vi "Apply.vi"(8 "Error In":errorcluster, 11 "Acquire Continuous Waveform CFG":refnum<class "Continuous Waveform Acq CFG.lvclass">) -> (0 "Error Out":errorcluster, 3 "Acquire Continuous Waveform CFG out":refnum<class "Continuous Waveform Acq CFG.lvclass">)   [LabVIEW 2023, in "RIGOL DS1054.lvlib" / "Continuous Waveform Acq CFG.lvclass"]
uses:
  Continuous Waveform Acq CFG.lvclass
  Continuous Waveform Acq CFG.lvclass/Continuous Waveform Acq CFG.ctl
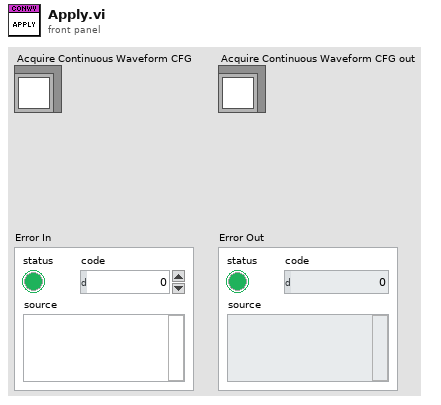
[diagram p1: front panel]
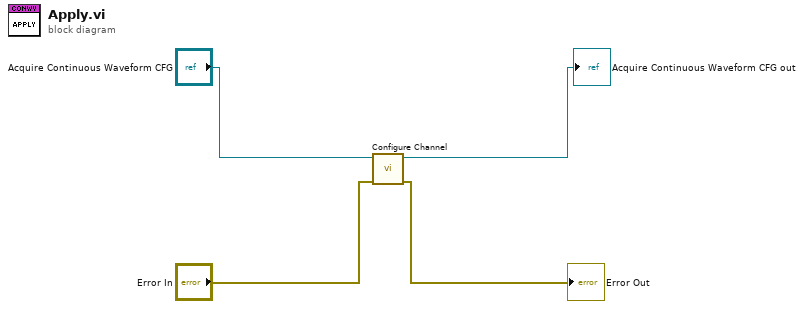
[diagram p0: block diagram]
diagram:
  n1 = call-dynamic "Configure Channel.vi"("error in"="Error In", "Continuous Waveforn Acq CFG in"="Acquire Continuous Waveform CFG") -> ("error out"=→"Error Out":errorcluster, "Continuous Waveforn Acq CFG out"=→"Acquire Continuous Waveform CFG out":refnum<class "Continuous Waveform Acq CFG.lvclass">)  [unwired: 8 in]
